vi "MT Apply Matched Filter (Generic).vi"(0 "input complex waveform":T1={"t0"=0.0, "dt"=1.0, "Y"=[]} {"Y" format="%.3f"; "dt" format="%^.2e"; "t0" format="%.4f"}, 5 "matched filter coefficients":dbl[](array[numeric]) format="%^.2e", 7 "samples per symbol (16)":i32=16, 11 "error in (no error)":errorcluster, 13 "reset? (T)":bool=TRUE) -> (4 "output complex waveform":T1 {"Y" format="%.3f"; "dt" format="%^.2e"; "t0" format="%.4f"}, 15 "error out":errorcluster)   [LabVIEW 2020, in "niDMT.lvlib"]
doc: "This polymorphic instance applies a matched filter to a PAM, ASK, QAM, and PSK-modulated input waveform."
uses:
  <vilib>/addons/Modulation/niDMT.lvlib
  <vilib>/addons/Modulation/Analog/controls/Complex Data Waveform.ctl
  <vilib>/addons/Modulation/niAMT.lvlib
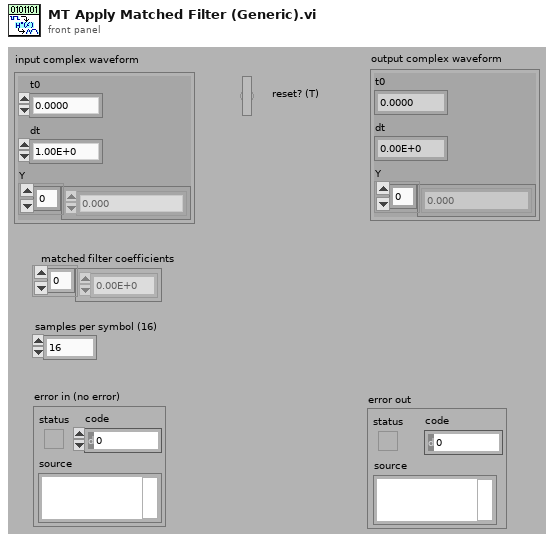
[diagram p1: front panel]
types:
  T1 = typedef "niAMT.lvlib/Complex Data Waveform.ctl" = cluster{"t0":dbl, "dt":dbl, "Y":cdb[]}
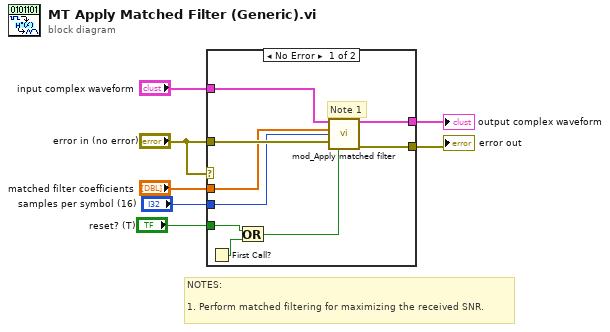
[diagram p0: block diagram]
diagram:
  # "NOTES:\n\n1. Perform matched filtering for maximizing the received SNR."
  n1 = case shown="No Error" "error in (no error)" {
    selector: "error in (no error)" -> [_ w17]
    tunnel: "error in (no error)" -> [w16 _]
    tunnel: "input complex waveform" -> [w15 _]
    tunnel: [w8 w17] -> w2
    tunnel: "matched filter coefficients" -> [w12 _]
    tunnel: "reset? (T)" -> [w14 _]
    tunnel: [w11 _] -> w3
    tunnel: "samples per symbol (16)" -> [w10 _]
    frame No Error {
      # "Note 1"
      n2 = First Call?() -> (First Call?: T/F=w13:bool)
      n3 = Or(x=w14, y=w13) -> (x .or. y?=w9:bool)
      n4 = call <vilib>:"mod_Apply matched filter.vi"("input complex waveform"=w15, "matched filter coefficients"=w12, "samples per symbol (16)"=w10, "error in (no error)"=w16, "reset? (T)"=w9) -> ("output complex waveform"=w11:T1, "error out"=w8:errorcluster)  [unwired: 9 out]
    }
    frame Error {
    }
  }
  "output complex waveform" <- w3
  "error out" <- w2
